vi "ExecutingCalibration.vi"(8 "error in (no error)":errorcluster, 10 "calibration_id":i32, 11 "ByteGSAPIBase in":refnum<class "ByteGSAPIBase.lvclass">) -> (0 "error out":errorcluster, 2 "Cluster":T1={"strumento_riferimento"={"id"=0, "nome"=""}, "controls"=[], "temperatura_c"=25.0, "umidita"=80.0} {"umidita" format="%.1g"; "temperatura_c" format="%.1g"; "controls"."incertezza" format="%.1g"; "controls"."deviazione_standard" format="%.1g"; "controls"."mpe_min" format="%.1g"; "controls"."mpe_max" format="%.1g"; "controls"."riferimento_obiettivo" format="%.1g"}, 3 "ByteGSAPIBase out":refnum<class "ByteGSAPIBase.lvclass">)   [LabVIEW 2019, in "ByteGSWebAPI.lvlib" / "ByteGSAPIBase.lvclass"]
uses:
  ByteGSAPIBase.lvclass
  BodyCalibrazioneMisure.ctl
  <vilib>/Bytelabs/ByteREST/ByteRESTClass/ByteRESTBase/HTTP/Status_Code.ctl
  ByteGSAPIBase.lvclass/ByteGSAPIBase.ctl
  <vilib>/Bytelabs/ByteREST/ByteRESTClass/ByteRESTBase/RESTBase.lvclass
  ByteGSWebAPI.lvlib
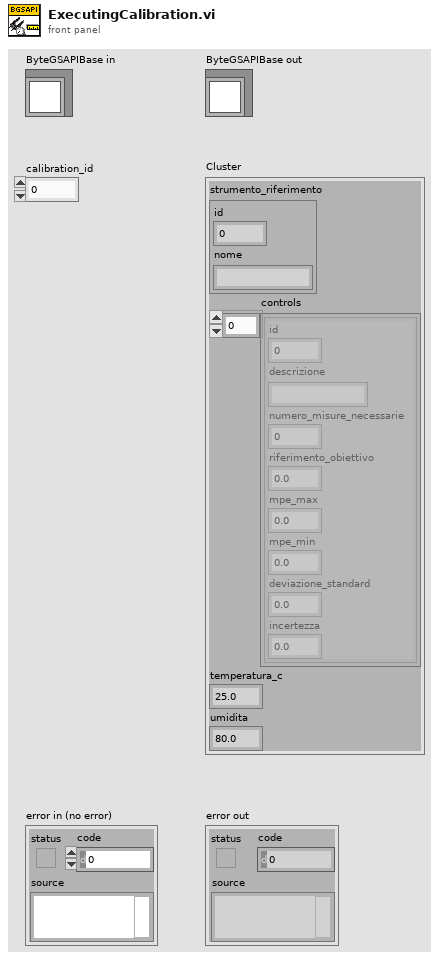
[diagram p1: front panel]
types:
  T1 = typedef "ByteGSWebAPI.lvlib/BodyCalibrazioneMisure.ctl" = cluster{"strumento_riferimento":cluster{"id":u16, "nome":string}, "controls":cluster{"id":u16, "descrizione":string, "numero_misure_necessarie":u16, "riferimento_obiettivo":dbl, "mpe_max":dbl, "mpe_min":dbl, "deviazione_standard":dbl, "incertezza":dbl}[], "temperatura_c":dbl, "umidita":dbl}
  T2 = typedef "ByteREST.lvlib/RESTBase.lvclass/Status_Code.ctl" = u16
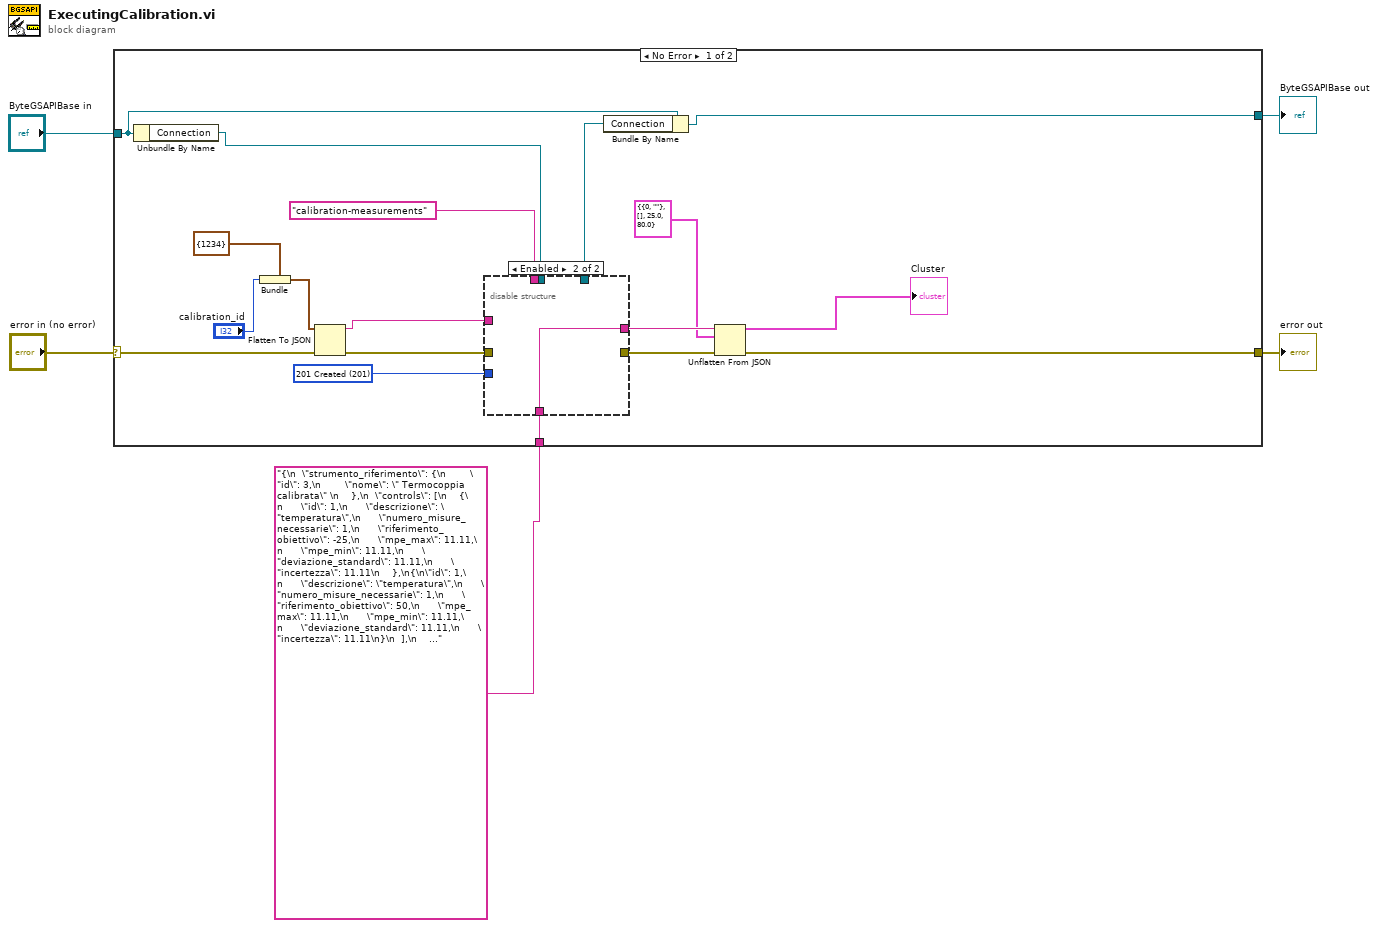
[diagram p0: block diagram]
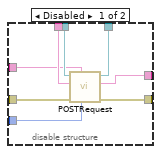
[diagram p2: hidden frame]
diagram:
  n1 = case shown="No Error" "error in (no error)" {
    selector: "error in (no error)" -> [w18 w34]
    tunnel: [w10 w34] -> w4
    tunnel: [w21 w33] -> w2
    tunnel: "ByteGSAPIBase in" -> [w23 w33]
    tunnel: "{\n  \"strumento_riferimento\": {\n        \"id\": 3,\n        \"nome\": \" Termocoppia calibrata\" \n    },\n  \"controls\": [\n    {\n      \"id\": 1,\n      \"descrizione\": \"temperatura\",\n      \"numero_misure_necessarie\": 1,\n      \"riferimento_obiettivo\": -25,\n      \"mpe_max\": 11.11,\n      \"mpe_min\": 11.11,\n      \"deviazione_standard\": 11.11,\n      \"incertezza\": 11.11\n    },\n{\n\"id\": 1,\n      \"descrizione\": \"temperatura\",\n      \"numero_misure_necessarie\": 1,\n      \"riferimento_obiettivo\": 50,\n      \"mpe_max\": 11.11,\n      \"mpe_min\": 11.11,\n      \"deviazione_standard\": 11.11,\n      \"incertezza\": 11.11\n}\n  ],\n    \"temperatura_c\": 25.0,\n    \"umidita\": 80.0\n}" -> [w6 _]
    frame No Error {
      w15 = T2 201 items=["200 OK"=200, "201 Created"=201, "400 Bad Request"=400, "401 Unauthorized"=401, "403 Forbidden"=403, "404 Not Found"=404, "405 Method Not Allowed"=405, "406 Not Acceptable"=406, "500 Internal Server Error"=500] ("expected response")
      n2 = Unbundle By Name(w23) -> ("Connection"=w22:refnum<class "RESTBase.lvclass">)
      n3 = Bundle(cluster=cluster{"calibration_id":i32} {"calibration_id"=1234}, "calibration_id"="calibration_id") -> (w7:cluster{"calibration_id":i32})
      n4 = Flatten To JSON(anything=w7, error in (no error)=w18) -> (JSON string=w13:string, 11:w14:errorcluster)  [unwired: 1 in]
      n5 = disable-structure shown="Enabled" {
        disable-tunnel: w22 -> [w31 _]
        disable-tunnel: [w30 _] -> w20
        disable-tunnel: "calibration-measurements" ("Request") -> [w29 _]
        disable-tunnel: [w28 w32] -> w17
        disable-tunnel: [w27 _] -> w16
        disable-tunnel: w15 -> [w26 _]
        disable-tunnel: w14 -> [w25 _]
        disable-tunnel: w13 -> [w24 _]
        disable-tunnel: w6 -> [_ w32]
        frame Disabled {
          n6 = call-dynamic "POSTRequest.vi"("expected response"=w26, "Body in"=w24, "error in (no error)"=w25, "Request"=w29, "ByteRESTBase in"=w31) -> ("error out"=w27:errorcluster, "Body"=w28:string, "ByteRESTBase out"=w30:refnum<class "RESTBase.lvclass">)  [unwired: 3 in, 1 out]
        }
        frame Enabled {
        }
      }
      n7 = Bundle By Name(cluster=w23, "Connection"=w20) -> (w21:refnum<class "ByteGSAPIBase.lvclass">)
      n8 = Unflatten From JSON(JSON string=w17, type and defaults=T1 {"strumento_riferimento"={"id"=0, "nome"=""}, "controls"=[], "temperatura_c"=25.0, "umidita"=80.0} ("Cluster 2"), error in (no error)=w16) -> (value=→"Cluster":T1, error out=w10:errorcluster)  [unwired: 4 in]
    }
    frame Error {
    }
  }
  "error out" <- w4
  "ByteGSAPIBase out" <- w2
